vi "Get Devices.vi"(8 "error in (no error)":errorcluster, 11 "DeviceManager in":refnum<class "DeviceManager.lvclass">) -> (0 "error out":errorcluster, 2 "Devices":refnum<class "Device.lvclass">[](array[class]), 3 "DeviceManager out":refnum<class "DeviceManager.lvclass">)   [LabVIEW 2020, in "PicoG-Core.lvlib" / "DeviceManager.lvclass"]
uses:
  DeviceManager.lvclass
  Device/Device.lvclass
  DeviceManager.lvclass/DeviceManager.ctl
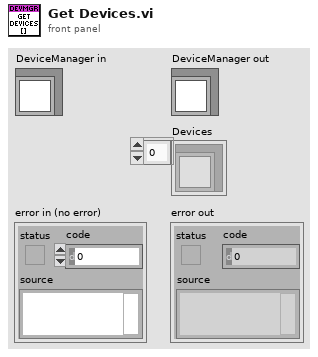
[diagram p1: front panel]
types:
  T1 = map{refnum<class "DeployResource.lvclass">, refnum<class "Device.lvclass">}
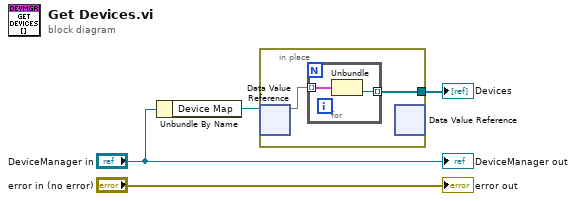
[diagram p0: block diagram]
diagram:
  n1 = Unbundle By Name("DeviceManager in") -> ("Device Map"=w2:refnum<data-value>)
  n2 = in-place {
    in-place-border: [w5] -> w1
    n3 = in-place-dvr #1(w2) -> (w6:T1)  [unwired: 1 out]
    n4 = for {
      tunnel: w6 -> [w8] mode=indexing
      tunnel: [w7] -> w5 mode=indexing
      n5 = Unbundle(w8) -> ("PicoG-Core:Device.lvclass"=w7:refnum<class "Device.lvclass">)  [unwired: 1 out]
    }
    n6 = in-place-dvr #1() -> ()  [unwired: 1 in, 2 out]
  }
  "Devices" <- w1
  "error out" <- "error in (no error)"
  "DeviceManager out" <- "DeviceManager in"
